vi "Test 1 Parallell Paths never cross.vi"(8 "error in (no error)":errorcluster, 11 "Test Case In":refnum<class "Vector Test.lvclass">) -> (0 "error out":errorcluster, 3 "Test Case Out":refnum<class "Vector Test.lvclass">)   [LabVIEW 2021, in "Vector Test.lvclass"]
uses:
  Vector Test.lvclass
  C:/Program Files (x86)/National Instruments/LabVIEW 2021/vi.lib/Astemes/LUnit/Test Case.lvclass
  <vilib>/Astemes/LUnit/Test Case.lvclass/Test Case.ctl
  <vilib>/Astemes/LUnit/Append Pass Result.vi
  <vilib>/Astemes/LUnit/Append Fail Result.vi
  Vector Test.lvclass/Vector Test.ctl
  Vector/Vector.lvclass
  <vilib>/Astemes/LUnit/Test Case.lvclass
  C:/Program Files (x86)/National Instruments/LabVIEW 2021/vi.lib/Astemes/LUnit/LUnit Runnable.lvclass
  C:/git/aoc-2023/Day 24/Vector Test/Vector Test.lvclass
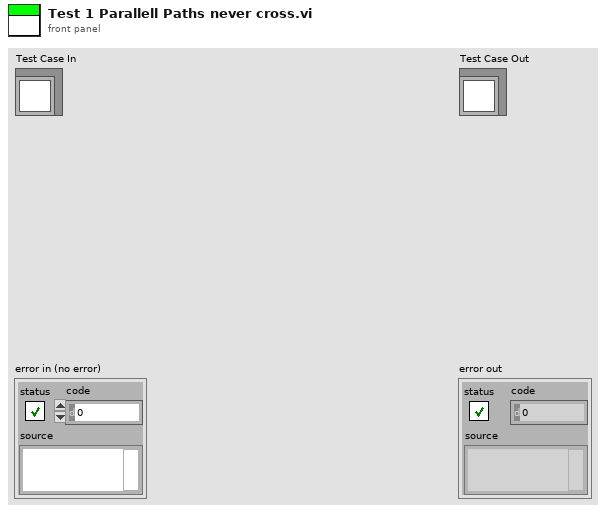
[diagram p1: front panel]
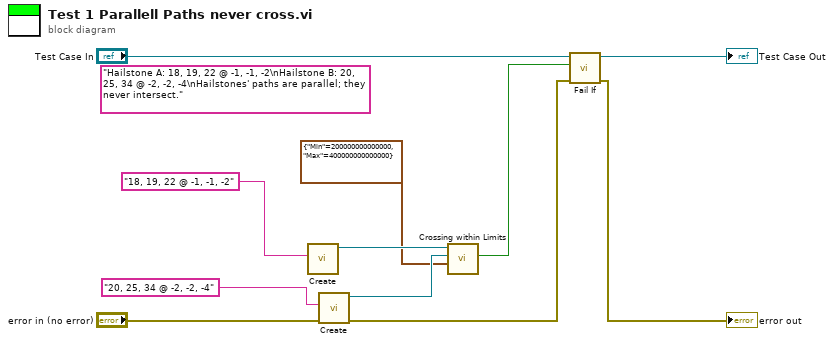
[diagram p0: block diagram]
diagram:
  (unwired) "Hailstone A: 18, 19, 22 @ -1, -1, -2\nHailstone B: 20, 25, 34 @ -2, -2, -4\nHailstones' paths are parallel; they never intersect." ("Input")
  n1 = call "Create.vi"("Input"="18, 19, 22 @ -1, -1, -2") -> ("Hailstone Out"=w4:refnum<class "Vector.lvclass">)  [unwired: 9 in, 1 out]
  n2 = call "Create.vi"("error in (no error)"="error in (no error)", "Input"="20, 25, 34 @ -2, -2, -4") -> ("error out"=w7:errorcluster, "Hailstone Out"=w3:refnum<class "Vector.lvclass">)  [unwired: 8 in]
  n3 = call "Crossing within Limits.vi"("Limits"=cluster{"Min":i64, "Max":i64} {"Min"=200000000000000, "Max"=400000000000000}, "Vector 2"=w3, "Vector In"=w4) -> ("Crossing?"=w2:bool)  [unwired: 6 in, 2 out]
  n4 = call <vilib>:"Fail If.vi"("error in (no error)"=w7, "Fail?"=w2, "LUnit Test Case In"="Test Case In") -> ("error out"=→"error out":errorcluster, "LUnit Test Case Out"=→"Test Case Out":refnum<class "Vector Test.lvclass">)  [unwired: 7 in]
